vi "XY Graph Load Single Column Plot from ASCII.vi"(4 "Default X step (1)":dbl=1.0, 6 "Default X start (0)":dbl, 8 "error in (no error)":errorcluster, 9 "Delimiter (TAB)":string="\t", 11 "String Array":string[](array[string])) -> (0 "error out":errorcluster, 1 "Single Column?":bool, 2 "Plot Array":cluster{"Array":dbl[], "Array":dbl[]}[](array[cluster]), 3 "String Array dup":string[](array[string]))   [LabVIEW 2021, in "XY Graph Add-Ons.lvlib"]
uses:
  XY Graph Add-Ons.lvlib
  f4805778-29b8-4bbd-bd65-a5295f137261.vi
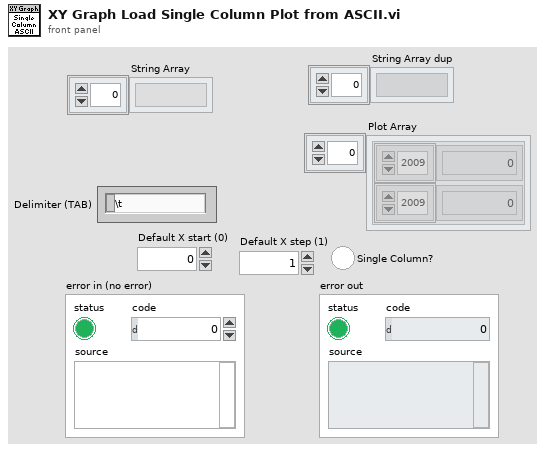
[diagram p1: front panel]
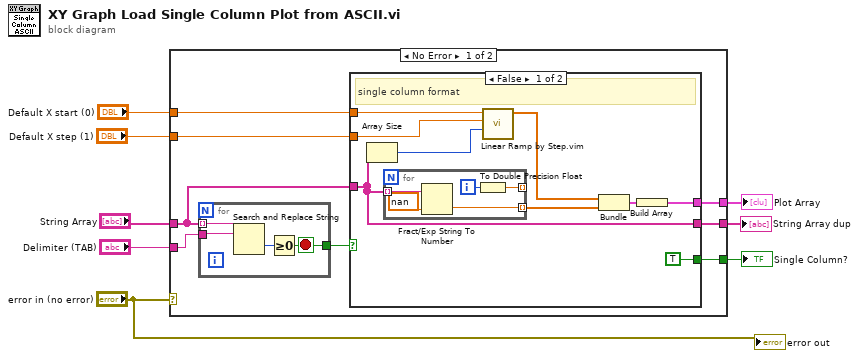
[diagram p0: block diagram]
diagram:
  n1 = case shown="No Error" "error in (no error)" {
    tunnel: "Delimiter (TAB)" -> [w16 _]
    tunnel: [w15 _] -> w7
    tunnel: [w14 _] -> w6
    tunnel: "String Array" -> [w13 w36]
    tunnel: [w12 w36] -> w3
    tunnel: "Default X step (1)" -> [w10 _]
    tunnel: "Default X start (0)" -> [w9 _]
    frame No Error {
      n2 = for {
        tunnel: w16 -> [w20]
        tunnel: w13 -> [w19] mode=indexing
        tunnel: [w17] -> w11
        stop <- w17 stop-if-true
        n3 = Search and Replace String(input string=w19, search string=w20) -> (offset past replacement=w18:i32)  [unwired: 6 in, 3 out]
        n4 = Greater Or Equal To 0?(x=w18) -> (x >= 0?=w17:bool)
      }
      n5 = case shown="False" w11 {
        tunnel: w13 -> [w22 w35]
        tunnel: [w27 _] -> w15
        tunnel: [TRUE ("Single Column?") _] -> w14
        tunnel: [w22 w35] -> w12
        tunnel: w10 -> [w25 _]
        tunnel: w9 -> [w23 _]
        frame False {
          # "single column format"
          n6 = Array Size(array=w22) -> (size(s)=w21:i32)
          n7 = for {
            tunnel: w22 -> [w34] mode=indexing
            tunnel: [w32] -> w28 mode=indexing
            tunnel: [w30] -> _ mode=indexing
            i -> [w31]
            n8 = Fract/Exp String To Number(string=w34, default (0 dbl)=nan ("default (0 DBL)")) -> (number=w32:dbl)  [unwired: 2 in, 1 out]
            n9 = To Double Precision Float(number=w31) -> (double precision float=w30:dbl)
          }
          n10 = call "Linear Ramp by Step.vim"("# Elements (1)"=w21, "Step (1)"=w25, "Start (0)"=w23) -> ("Ramp"=w24:dbl[])  [unwired: 8 in]
          n11 = Bundle("Ramp"=w24, w28) -> (w29:cluster{"Ramp":dbl[], dbl[]})  [unwired: 1 in]
          n12 = Build Array(w29) -> (w27:cluster{"Ramp":dbl[], dbl[]}[])
        }
        frame True {
          # "not a single column file"
        }
      }
    }
    frame Error {
    }
  }
  "Plot Array" <- w7
  "Single Column?" <- w6
  "String Array dup" <- w3
  "error out" <- "error in (no error)"
